vi "ExCircNframeBigBufBin2x.vi"() -> ()   [LabVIEW 2010]
panel:
  out "ready to \nstart":bool
  in  "Start collection":bool
  in  "Timing Mode":u32(ring)=1 items=["N/A", "Timed Mode/Free run", "Trigger First (only PM)", "Strobed/Ext Sync", "Bulb Mode (PM only)", "Variable Timed mode (PM only)", "Flash Mode (only some PM)"]
  in  "Number of Images":u32=1 min=1 step=1
  in  "Intensifier":bool
  in  "Temperature":dbl=-10.0 format="%.2f"
  in  "Exposure":dbl min=0.0 step=0.001 format="%.3f"
  out "error out":errorcluster
  in  "error in (no error)":errorcluster
  # "ExCircNframeBigBufBin2x:\nThis example collects, displays, and saves in \na .spe file the number of images selected. This \nexample requires the camera have circular \nbuffers capability. \nFirst this example creates an array of image \nhandles. It then collects data into this array.\nFinally it displays and saves all the images."
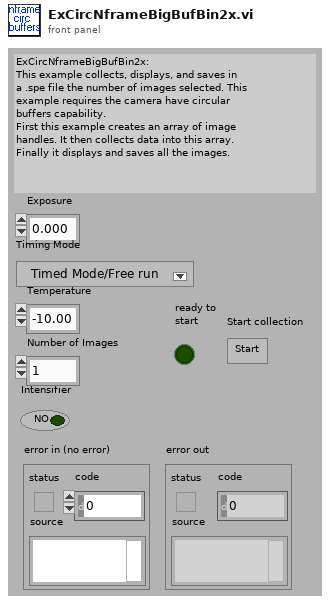
[diagram p1: front panel]
types:
  T1 = cluster{"acquire focus mode":u32, "Exposure":dbl, "Number of Images":u32, "Software accumulation":u32}
  T2 = cluster{"Camera Handle":u32, "Pulser Handle":u32, "File Handle":u32, "Display Handle":u32, "Image Handle":u32}
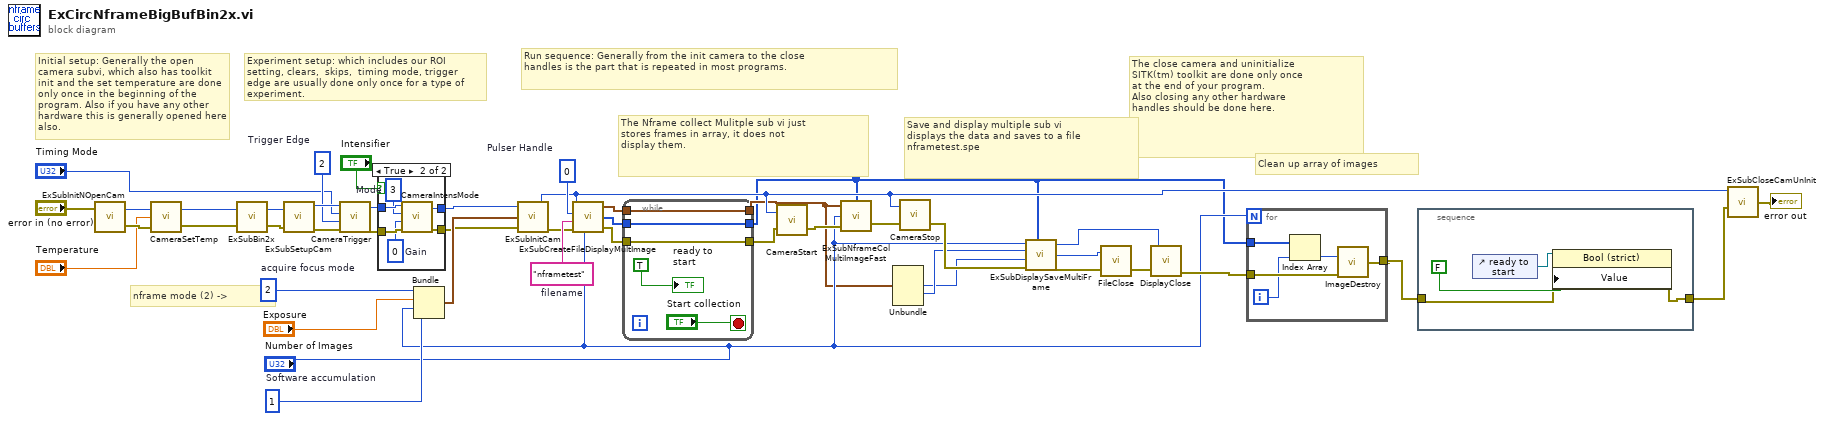
[diagram p0: block diagram]
diagram:
  w35 = u32 0  # Pulser Handle
  w36 = u32 2  # Trigger Edge
  w38 = u32 2  # acquire focus mode
  w37 = u32 1  # Software accumulation
  w45 = "nframetest"  # filename
  # "Clean up array of images"
  # "Save and display multiple sub vi\ndisplays the data and saves to a file\nnframetest.spe"
  # "The Nframe collect Mulitple sub vi just \nstores frames in array, it does not \ndisplay them."
  # "The close camera and uninitialize\nSITK(tm) toolkit are done only once\nat the end of your program.\nAlso closing any other hardware \nhandles should be done here."
  # "Run sequence: Generally from the init camera to the close \nhandles is the part that is repeated in most programs."
  # "Experiment setup: which includes our ROI setting, clears,  skips,  timing mode, trigger edge are usually done only once for a type of experiment."
  # "Initial setup: Generally the open camera subvi, which also has toolkit init and the set temperature are done only once in the beginning of the program. Also if you have any other hardware this is generally opened here also."
  # "nframe mode (2) ->"
  n1 = call "ExSubInitNOpenCam.vi"("error in (no error)"="error in (no error)") -> ("Camera Handle"=w26:u32, "error out"=w25:errorcluster)
  n2 = call <userlib>:"CameraSetTemp.vi"("error in (no error)"=w25, "Temperature"="Temperature", "Camera Handle"=w26) -> ("error out"=w28:errorcluster, "Camera Handle"=w27:u32)
  n3 = call "ExSubBin2x.vi"("error in (no error)"=w28, "Camera Handle"=w27) -> ("error out"=w22:errorcluster, "Camera Handle"=w23:u32)
  n4 = call "ExSubSetupCam.vi"("error in (no error)"=w22, "Camera Handle"=w23) -> ("error out"=w39:errorcluster, "Camera Handle"=w40:u32)
  n5 = call <userlib>:"CameraTrigger.vi"("error in"=w39, "Trigger Edge"=w36, "Timing Mode"="Timing Mode", "Camera Handle"=w40) -> ("error out"=w32:errorcluster, "Camera Handle"=w34:u32)
  n6 = case shown="True" "Intensifier" {
    tunnel: w34 -> [w47 w53]
    tunnel: [w47 w52] -> w33
    tunnel: w32 -> [w46 w51]
    tunnel: [w46 w50] -> w31
    frame False {
    }
    frame True {
      w48 = u32 0  # Gain
      w49 = u32 3  # Mode
      n7 = call <userlib>:"CameraIntensMode.vi"("error in"=w51, "Intensifier Gain"=w48, "Mode"=w49, "Camera Handle"=w53) -> ("error out"=w50:errorcluster, "Camera Handle"=w52:u32)
    }
  }
  n8 = Bundle("acquire focus mode"=w38, "Exposure"="Exposure", "Number of Images"="Number of Images", "Software accumulation"=w37) -> (w42:T1)  [unwired: 1 in]
  n9 = call "ExSubInitCam.vi"("error in (no error)"=w31, "Camera Information"=w42, "Camera Handle"=w33) -> ("error out"=w41:errorcluster, "Camera Handle"=w20:u32)
  n10 = call "ExSubCreateFileDisplayMultImage.vi"("Camera Handle"=w20, "Pulser Handle"=w35, "File and Display Name"=w45, "error in (no error)"=w41, "Number of Images"="Number of Images") -> ("Handles Out"=w8:T2, "Array"=w4:u32[], "error out"=w6:errorcluster)
  n11 = while {
    tunnel: w8 -> [w58]
    tunnel: [w58] -> w7
    tunnel: w6 -> [w57]
    tunnel: [w57] -> w5
    tunnel: w4 -> [w56]
    tunnel: [w56] -> w3
    stop <- "Start collection" stop-if-true
    "ready to \nstart" <- TRUE
  }
  n12 = call <userlib>:"CameraStart.vi"("error in"=w5, "Camera Handle"=w20) -> ("error out"=w29:errorcluster)  [unwired: 1 out]
  n13 = call "ExSubNframeColMultiImageFast.vi"("image handles"=w3, "error in (no error)"=w29, "Number of Images"="Number of Images", "Handle Cluster"=w7) -> ("error out"=w21:errorcluster)  [unwired: 1 out]
  n14 = Unbundle(w7) -> ("File Handle"=w15:u32, "Display Handle"=w16:u32)  [unwired: 3 out]
  n15 = call <userlib>:"CameraStop.vi"("error in"=w21, "Camera Handle"=w20) -> ("error out"=w17:errorcluster)  [unwired: 1 out]
  n16 = call "ExSubDisplaySaveMultiFrame.vi"("Number of Images"="Number of Images", "Display Handle"=w16, "file handle"=w15, "error in (no error)"=w17, "Data handles"=w3) -> ("Display Handle"=w10:u32, "file Handle"=w11:u32, "error out"=w12:errorcluster)
  n17 = call <userlib>:"FileClose.vi"("error in"=w12, "File Handle"=w11) -> ("error out"=w14:errorcluster)
  n18 = call <userlib>:"DisplayClose.vi"("error in"=w14, "Display Handle"=w10) -> ("error out"=w13:errorcluster)
  n19 = for {
    N: "Number of Images" -> [_]
    tunnel: w13 -> [w63]
    tunnel: [w62] -> w2
    tunnel: w3 -> [w60]
    i -> [w61]
    n20 = Index Array(array=w60, index=w61) -> (element=w59:u32)
    n21 = call <userlib>:"ImageDestroy.vi"("error in"=w63, "Data handle"=w59) -> ("error out"=w62:errorcluster)
  }
  n22 = stacked-sequence {
    tunnel: w2 -> [w65]
    tunnel: [w64] -> w1
    frame #0 {
      n23 = control-ref of="ready to \nstart"() -> (w67:refnum<vi>)
      n24 = property class="Bool (strict)"(reference=w67, error in=w65, "Value"=FALSE) -> (error out=w64:errorcluster)  [unwired: 1 out]
    }
  }
  n25 = call "ExSubCloseCamUnInit.vi"("error in (no error)"=w1, "Camera Handle"=w20) -> ("error out"=→"error out":errorcluster)
